vi "Variant to String.vi"(8 "error in":errorcluster, 11 "Variant":variant) -> (0 "error out":errorcluster, 2 "type":T1, 3 "Output string":string)   [LabVIEW 2020]
uses:
  <vilib>/Utility/Data Type/Type Definitions/Data Type.ctl
  <vilib>/Utility/Data Type/NI_Data Type.lvlib
panel:
  out "double precision float":dbl
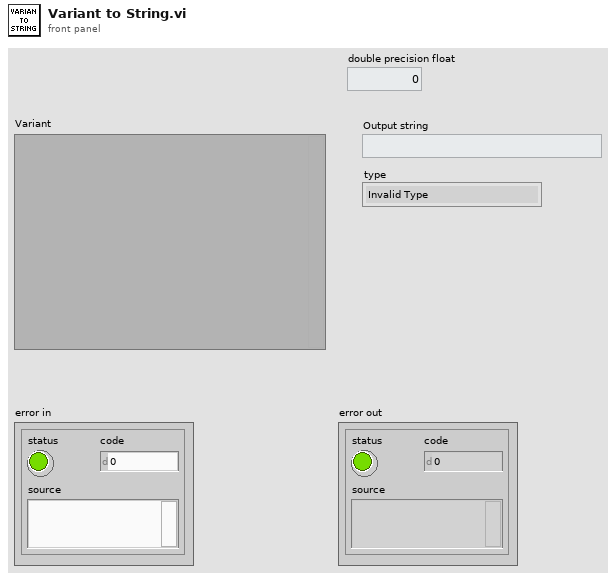
[diagram p1: front panel]
types:
  T1 = typedef "NI_Data Type.lvlib/Data Type.ctl" = enum8{"Invalid Type", "Void", "I8", "I16", "I32", "I64", "U8", "U16", "U32", "U64", "Single Float", "Double Float", "Extended Float", "Single Complex", "Double Complex", "Extended Complex", "Enum U8", "Enum U16", "Enum U32", "Enum U64", "Single Float With Unit", "Double Float With Unit", "Extended Float With Unit", "Single Complex with Unit", "Double Complex with Unit", "Extended Complex with Unit", "Boolean", "String", "Path", "Picture", "Tag", "Array", "Cluster", "Variant", "LV Variant", "Waveform", "Timestamp", "Digital Waveform", "Digital Data", "ExpressData", "Refnum", "External Data", "VI", "Poly VI", "LabVIEW Class Instance", "Fixed Point", "Set Collection", "Map Collection"}
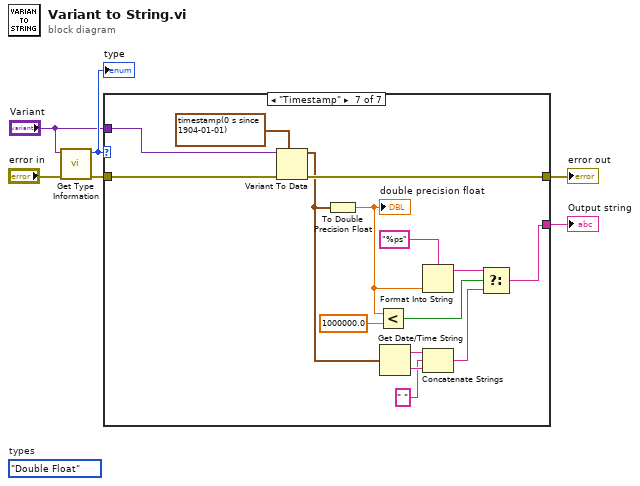
[diagram p0: block diagram]
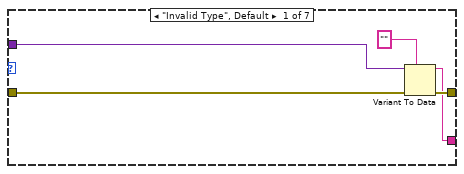
[diagram p2: hidden frame]
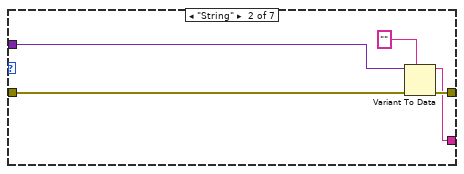
[diagram p3: hidden frame]
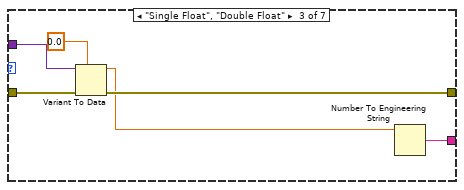
[diagram p4: hidden frame]
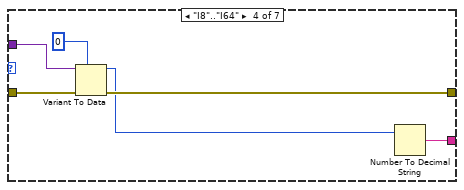
[diagram p5: hidden frame]
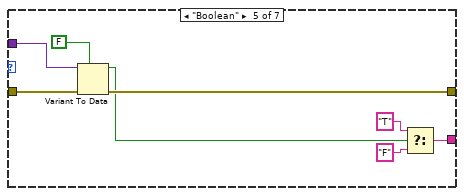
[diagram p6: hidden frame]
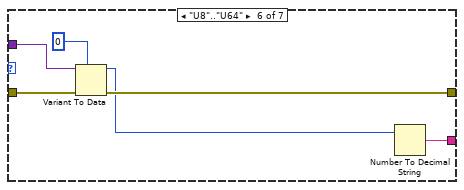
[diagram p7: hidden frame]
diagram:
  (unwired) Data_Type."Double Float"  # types
  n1 = call <vilib>:"Get Type Information.vi"("error in (no error)"="error in", "variant"="Variant") -> ("error out"=w4:errorcluster, "type"=w6:T1)  [unwired: 5 in, 3 out]
  "type" <- w6
  n2 = case shown="\"Timestamp\"" w6 {
    tunnel: w4 -> [w11 w16 w22 w28 w36 w42 w57]
    tunnel: [w10 w15 w21 w27 w35 w41 w56] -> w3
    tunnel: "Variant" -> [w8 w13 w19 w25 w33 w39 w54]
    tunnel: [w7 w12 w17 w23 w32 w37 w43] -> w1
    frame "Invalid Type", Default {
      n3 = Variant To Data(error in=w11, type="", Variant=w8) -> (data=w7:string, error out=w10:errorcluster)
    }
    frame "String" {
      n4 = Variant To Data(error in=w16, type="", Variant=w13) -> (data=w12:string, error out=w15:errorcluster)
    }
    frame "Single Float", "Double Float" {
      n5 = Variant To Data(error in=w22, type=0.0, Variant=w19) -> (data=w18:dbl, error out=w21:errorcluster)
      n6 = Number To Engineering String(4:w18) -> (0:w17:string)  [unwired: 3 in]
    }
    frame "I8".."I64" {
      n7 = Variant To Data(error in=w28, type=i64 0, Variant=w25) -> (data=w24:i64, error out=w27:errorcluster)
      n8 = Number To Decimal String(number=w24) -> (decimal integer string=w23:string)  [unwired: 1 in]
    }
    frame "Boolean" {
      n9 = Variant To Data(error in=w36, type=FALSE, Variant=w33) -> (data=w31:bool, error out=w35:errorcluster)
      n10 = Select(t="T", s=w31, f="F") -> (s? t:f=w32:string)
    }
    frame "U8".."U64" {
      n11 = Variant To Data(error in=w42, type=u64 0, Variant=w39) -> (data=w38:u64, error out=w41:errorcluster)
      n12 = Number To Decimal String(number=w38) -> (decimal integer string=w37:string)  [unwired: 1 in]
    }
    frame "Timestamp" {
      n13 = Variant To Data(error in=w57, type=timestamp(0 s since 1904-01-01), Variant=w54) -> (data=w50:timestamp, error out=w56:errorcluster)
      n14 = To Double Precision Float(number=w50) -> (double precision float=w45:dbl)
      "double precision float" <- w45
      n15 = Less?(x=w45, y=1000000.0) -> (x < y?=w48:bool)
      n16 = Get Date/Time String(seconds (now)=w50) -> (date string=w53:string, time string=w52:string)  [unwired: 2 in]
      n17 = Format Into String(format string="%ps", w45) -> (resulting string=w46:string)  [unwired: 2 in, 1 out]
      n18 = Concatenate Strings(w53, " " ("string"), w52) -> (w47:string)
      n19 = Select(t=w46, s=w48, f=w47) -> (s? t:f=w43:string)
    }
  }
  "error out" <- w3
  "Output string" <- w1
